vi "OE2031&OE2041_Configure Sine Out.vi"(7 "OE2041_Configure Sine Out":T1={"Start Value(V)"=0.1, "Sine Output Amplitude (V)"=1.0, "Stop Valve(V)"=1.0, "Sine Step Valve(V)"=0.1, "Step Time(ms) "=1000, "Sine Step Percent(%)"=10.0, "SineOut Mode"=0, "Sine Run Mode"=0, "ADD Mode"=0} {"ADD Mode" items=["OFF", "ON"]; "Sine Run Mode" items=["Stop", "Single", "Loop"]; "SineOut Mode" items=["OFF", "Fixed", "Linear", "Log"]; "Sine Step Percent(%)" min=0.0 max=100.0 format="%#.2g"; "Step Time(ms)" min=1 max=100000; "Sine Step Valve(V)" min=1e-06 max=1.0 format="%#.3g"; "Stop Valve(V)" min=1e-06 max=1.0 format="%#.3g"; "Sine Output Amplitude (V)" min=1e-06 max=1.0 format="%#.3g"; "Start Value(V)" min=1e-06 max=1.0 format="%#.3g"}, 8 "Error in (no error)":errorcluster caption="error out（no error）", 9 "Remote Mode":u16(ring) items=["USB"=0, "RS232"=1, "Ethernet"=3], 10 "Connection ID in":refnum<k5>, 11 "VISA resource name":refnum<visa-resource-name>) -> (0 "Error out":errorcluster caption="error out", 1 "Output String":string, 2 "Connection ID out":refnum<k5>, 3 "VISA resource  out":refnum<visa-resource-name>)   [LabVIEW 2011]
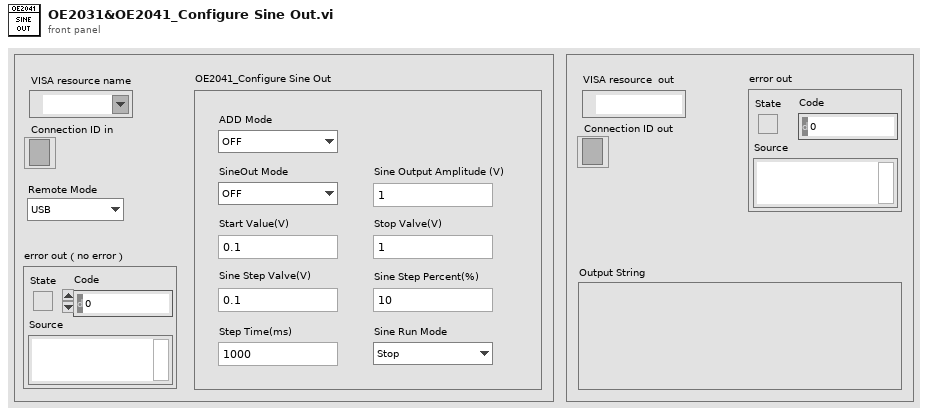
[diagram p1: front panel]
types:
  T1 = cluster{"Start Value(V)":dbl, "Sine Output Amplitude (V)":dbl, "Stop Valve(V)":dbl, "Sine Step Valve(V)":dbl, "Step Time(ms) ":u32, "Sine Step Percent(%)":dbl, "SineOut Mode":u8, "Sine Run Mode":u8, "ADD Mode":u8}
  T2 = enum16{"ISRC", "IGND", "ICPL", "ILIN", "PHAS", "FMOD", "RSLP", "FREQ", "SWPT", "SLLM", "SULM", "SSLL", "SSLG", "STLM", "SWRM", "IRNG", "SENS", "RMOD", "OFLT", "OFSL", "SYNC", "DMOD", "HARM", "DARB", "SWVT", "SLVL", "SVLL", "SVUL", "SVSL", "SVSG", "SVTM", "SVRM", "RALL", "SNAP", "OUTP", "OAUX", "COUT", "CAUX", "COFP", "CEXP", "FPOP", "OEXP", "*IDN", "*RST", "OVLD", "INOV", "GNOV", "*PLL", "SSET", "RSET", "AGAN", "APHS", "ARSV", "ASCL", "EQCD", "EQCS", "SPED", "SRAT", "SLEN", "SSLE", "STRG", "SPRM", "STRD", "PAUS", "REST", "SPTS", "TRCA", "TEMP", "RSTU", "IHNZ", "DEQU", "SADD", "ARNG", "CSPE", "ISRCD", "IGNDD", "ICPLD", "ILIND", "PHASD", "FMODD", "RSLPD", "FREQD", "SWPTD", "SLLMD", "SULMD", "SSLLD", "SSLGD", "STLMD", "SWRMD", "SENSD", "RMODD", "OFLTD", "OFSLD", "SYNCD", "HARMD", "EQCDD", "EQCSD", "SNAPD", "OUTPD", "SWVTD", "SLVLD", "SVLLD", "SVULD", "SVSLD", "SVSGD", "SVTMD", "SVRMD", "SVDCD", "ARSVD", "AGAND", "APHSD", "ASCLD", "FPOPD", "CAUXD", "OEXPD", "SPEDD", "SRATD", "SLEND", "SSLED", "STRGD", "SPRMD", "STRDD", "PAUSD", "RESTD", "SPTSD", "TRCAD", "*IDND", "*RSTD", "INOVD", "GNOVD", "*PLLD", "SSETD", "RSETD", "RALLD"}
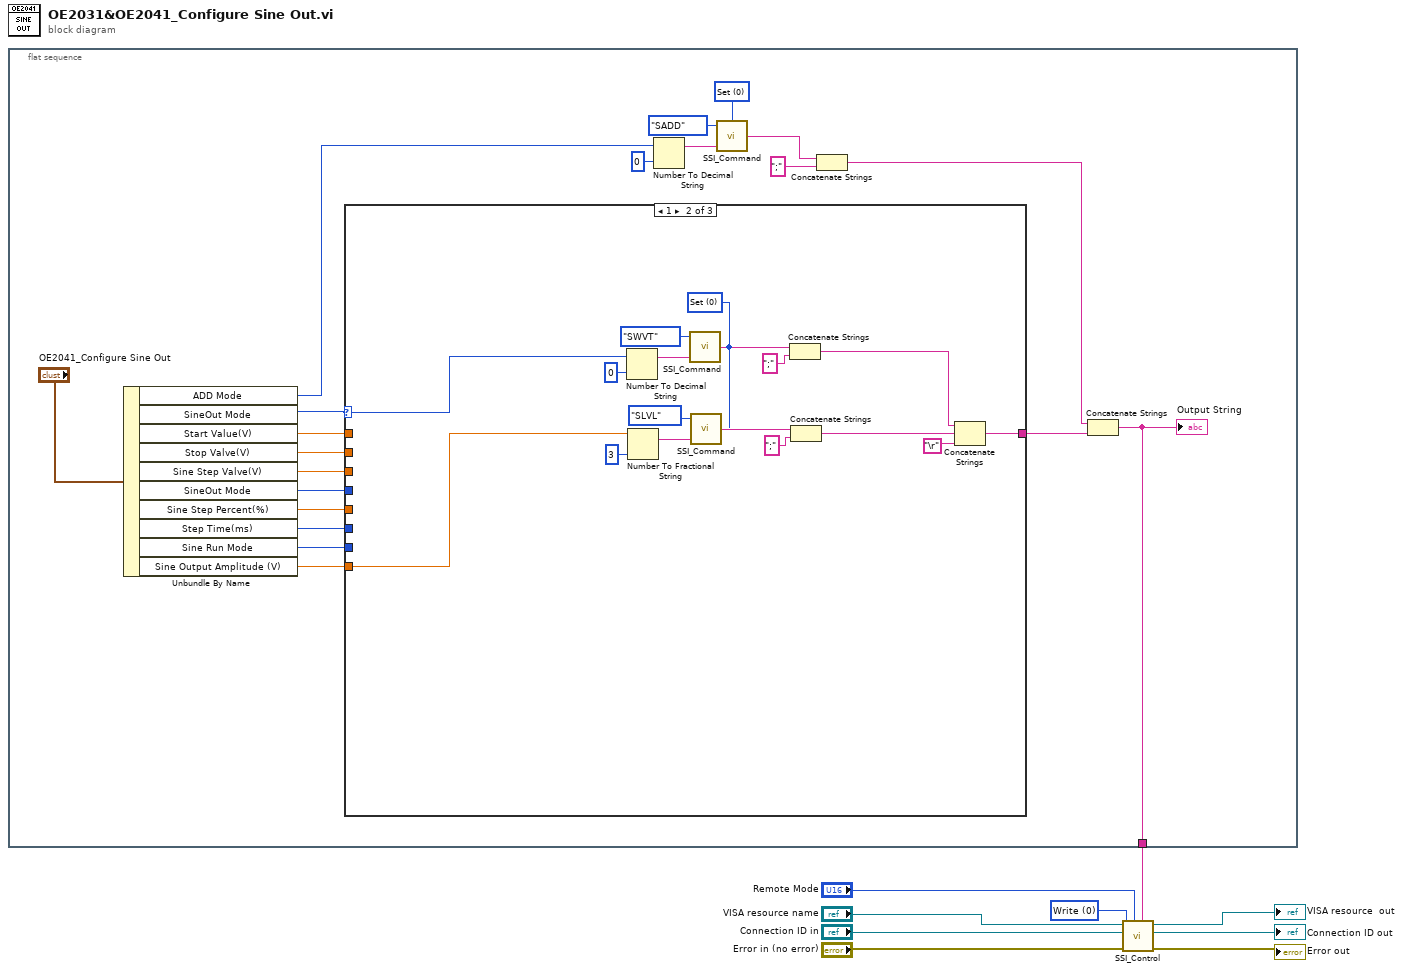
[diagram p0: block diagram]
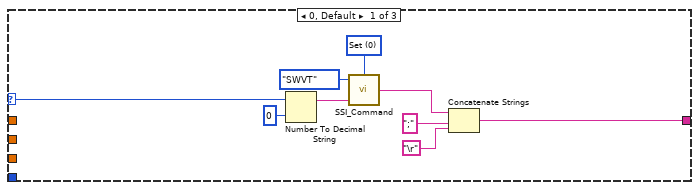
[diagram p2: hidden frame]
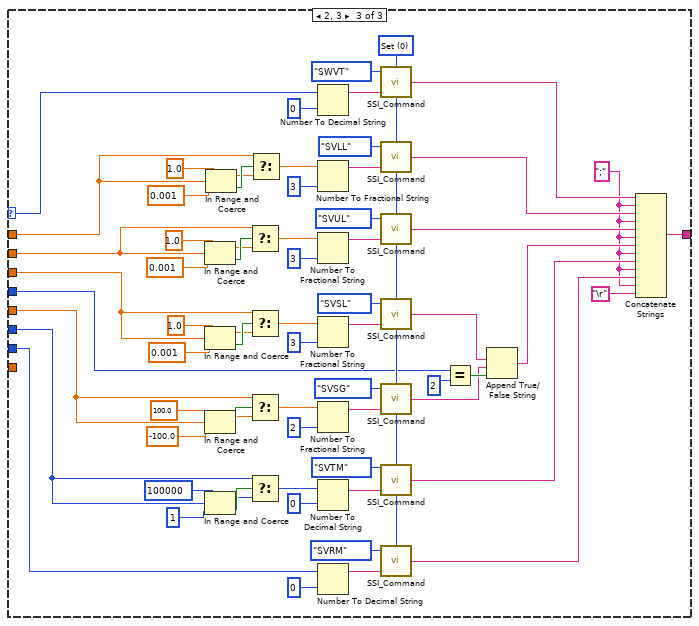
[diagram p3: hidden frame]
diagram:
  w7 = u16 0 items=["Write", "Read"] ("Control")
  n1 = flat-sequence {
    tunnel: [w12] -> w1
    frame #0 {
      w17 = u16 0 items=["Set", "Query"] ("Opera")
      n2 = Unbundle By Name("OE2041_Configure Sine Out") -> ("ADD Mode"=w14:u8, "SineOut Mode"=w21:u8, "Start Value(V)"=w28:dbl, "Stop Valve(V)"=w27:dbl, "Sine Step Valve(V)"=w26:dbl, "SineOut Mode"=w24:u8, "Sine Step Percent(%)"=w23:dbl, "Step Time(ms)"=w22:u32, "Sine Run Mode"=w25:u8, "Sine Output Amplitude (V)"=w10:dbl)
      n3 = case shown="1" w21 {
        selector: w21 -> [w31 w42 w63]
        tunnel: [w32 w43 w89] -> w13
        tunnel: w28 -> [_ _ w69]
        tunnel: w27 -> [_ _ w70]
        tunnel: w26 -> [_ _ w82]
        tunnel: w25 -> [_ _ w67]
        tunnel: w24 -> [_ _ w66]
        tunnel: w23 -> [_ _ w65]
        tunnel: w22 -> [_ _ w64]
        tunnel: w10 -> [_ w39 _]
        frame 0, Default {
          w35 = u16 0 items=["Set", "Query"] ("Opera")
          n4 = Number To Decimal String(number=w31, width (-)=i16 0 ("宽度(-)")) -> (decimal integer string=w37:string)
          n5 = call "SSI_Command.vi"("Opera"=w35, "Paramter"=w37, "Command Type"=T2."SWVT") -> ("Output string"=w36:string)  [unwired: 1 in]
          n6 = Concatenate Strings(w36, ";" ("替换字符串(\"\")"), "\r") -> (w32:string)
        }
        frame 1 {
          w49 = u16 0 items=["Set", "Query"] ("Opera")
          n7 = Number To Decimal String(number=w42, width (-)=i16 0 ("宽度(-)")) -> (decimal integer string=w51:string)
          n8 = Number To Fractional String(number=w39, precision (6)=i16 3 ("宽度(-)")) -> (F-format string=w54:string)  [unwired: 2 in]
          n9 = call "SSI_Command.vi"("Opera"=w49, "Paramter"=w51, "Command Type"=T2."SWVT") -> ("Output string"=w50:string)  [unwired: 1 in]
          n10 = call "SSI_Command.vi"("Opera"=w49, "Paramter"=w54, "Command Type"=T2."SLVL") -> ("Output string"=w53:string)  [unwired: 1 in]
          n11 = Concatenate Strings(w50, ";" ("替换字符串(\"\")")) -> (w44:string)
          n12 = Concatenate Strings(w53, ";" ("替换字符串(\"\")")) -> (w46:string)
          n13 = Concatenate Strings(w44, w46, "\r") -> (w43:string)
        }
        frame 2, 3 {
          w87 = ";"
          w100 = u16 0 items=["Set", "Query"] ("Opera")
          n14 = In Range and Coerce(upper limit=1.0 ("上限"), x=w70, lower limit=0.001 ("下限")) -> (coerced(x)=w80:dbl, In Range?=w81:bool)
          n15 = In Range and Coerce(upper limit=1.0 ("上限"), x=w82, lower limit=0.001 ("下限")) -> (coerced(x)=w85:dbl, In Range?=w86:bool)
          n16 = In Range and Coerce(upper limit=100.0 ("上限"), x=w65, lower limit=-100.0 ("下限")) -> (coerced(x)=w105:dbl, In Range?=w106:bool)
          n17 = In Range and Coerce(upper limit=u32 100000 ("上限"), x=w64, lower limit=u32 1 ("下限")) -> (coerced(x)=w109:u32, In Range?=w110:bool)
          n18 = In Range and Coerce(upper limit=1.0 ("上限"), x=w69, lower limit=0.001 ("下限")) -> (coerced(x)=w74:dbl, In Range?=w75:bool)
          n19 = Select(t=w70, s=w81, f=w80) -> (s? t:f=w77:dbl)
          n20 = Select(t=w82, s=w86, f=w85) -> (s? t:f=w76:dbl)
          n21 = Select(t=w65, s=w106, f=w105) -> (s? t:f=w98:dbl)
          n22 = Select(t=w64, s=w110, f=w109) -> (s? t:f=w99:u32)
          n23 = Select(t=w69, s=w75, f=w74) -> (s? t:f=w71:dbl)
          n24 = Number To Decimal String(number=w63, width (-)=i16 0 ("精度(6)")) -> (decimal integer string=w119:string)
          n25 = Number To Fractional String(number=w71, precision (6)=i16 3 ("精度(6)")) -> (F-format string=w117:string)  [unwired: 2 in]
          n26 = Number To Fractional String(number=w77, precision (6)=i16 3 ("精度(6)")) -> (F-format string=w115:string)  [unwired: 2 in]
          n27 = Number To Fractional String(number=w76, precision (6)=i16 3 ("精度(6)")) -> (F-format string=w113:string)  [unwired: 2 in]
          n28 = Number To Fractional String(number=w98, precision (6)=i16 2 ("精度(6)")) -> (F-format string=w111:string)  [unwired: 2 in]
          n29 = Number To Decimal String(number=w99, width (-)=i16 0 ("精度(6)")) -> (decimal integer string=w121:string)
          n30 = Number To Decimal String(number=w67, width (-)=i16 0 ("精度(6)")) -> (decimal integer string=w101:string)
          n31 = call "SSI_Command.vi"("Opera"=w100, "Paramter"=w119, "Command Type"=T2."SWVT") -> ("Output string"=w95:string)  [unwired: 1 in]
          n32 = call "SSI_Command.vi"("Opera"=w100, "Paramter"=w117, "Command Type"=T2."SVLL") -> ("Output string"=w94:string)  [unwired: 1 in]
          n33 = call "SSI_Command.vi"("Opera"=w100, "Paramter"=w115, "Command Type"=T2."SVUL") -> ("Output string"=w93:string)  [unwired: 1 in]
          n34 = call "SSI_Command.vi"("Opera"=w100, "Paramter"=w113, "Command Type"=T2."SVSL") -> ("Output string"=w96:string)  [unwired: 1 in]
          n35 = call "SSI_Command.vi"("Opera"=w100, "Paramter"=w111, "Command Type"=T2."SVSG") -> ("Output string"=w97:string)  [unwired: 1 in]
          n36 = call "SSI_Command.vi"("Opera"=w100, "Paramter"=w121, "Command Type"=T2."SVTM") -> ("Output string"=w91:string)  [unwired: 1 in]
          n37 = call "SSI_Command.vi"("Opera"=w100, "Paramter"=w101, "Command Type"=T2."SVRM") -> ("Output string"=w90:string)  [unwired: 1 in]
          n38 = Equal?(x=w66, y=u8 2 ("x")) -> (x = y?=w123:bool)
          n39 = Append True/False String(1:w123, 2:w97, 3:w96) -> (0:w92:string)  [unwired: 1 in]
          n40 = Concatenate Strings(w95, w87, w94, w87, w93, w87, w92, w87, w91, w87, w90, w87, "\r") -> (w89:string)
        }
      }
      n41 = Number To Decimal String(number=w14, width (-)=i16 0 ("宽度(-)")) -> (decimal integer string=w19:string)
      n42 = call "SSI_Command.vi"("Opera"=w17, "Paramter"=w19, "Command Type"=T2."SADD") -> ("Output string"=w18:string)  [unwired: 1 in]
      n43 = Concatenate Strings(w18, ";" ("替换字符串(\"\")")) -> (w11:string)
      n44 = Concatenate Strings(w11, w13) -> (w12:string)
      "Output String" <- w12
    }
  }
  n45 = call "SSI_Control.vi"("Write Buffer"=w1, "Remote Mode"="Remote Mode", "Error in (no error)"="Error in (no error)", "Control"=w7, "Connection ID in"="Connection ID in", "VISA resource name"="VISA resource name") -> ("Error out"=→"Error out":errorcluster, "Connection ID out"=→"Connection ID out":refnum<k5>, "VISA resource  out"=→"VISA resource  out":refnum<visa-resource-name>)  [unwired: 2 in, 1 out]
